vi "Update Clock Map.vi"(6 "Name":string, 7 "Reset":bool, 8 "error in (no error)":errorcluster, 9 "ClockID":u8, 10 "Timestamp Pair":T1, 11 "Clock History Map in":T3) -> (0 "error out":errorcluster, 3 "Clock History Map out":map{u8, T2}(c390))   [LabVIEW 2021, in "Time_CIF_U.lvlib"]
uses:
  Time_CIF_U.lvlib
  Typedef/Clock History Map.ctl
  Typedef/Clock History.ctl
  Typedef/Timestamp Pair.ctl
  Typedef/Errors.ctl
  <vilib>/Utility/miscctls.llb/LVMapReplaceAction.ctl
  <vilib>/Analysis/6fits.llb/Curve Fitting Criteria.ctl
  Errors/Append Error Location.vi
  <vilib>/Analysis/3filter.llb/Savitzky-Golay Filter.vi
  <vilib>/Analysis/3filter.llb/Savitzky-Golay Filter (DBL).vi
  <vilib>/Analysis/baseanly.llb/Std Deviation and Variance.vi
  <vilib>/Analysis/NI_AALPro.lvlib
  DataTypes/DataTypes_CIF_U.lvlib
panel:
  out "Slope":dbl
  out "XY Graph":cluster{i64[], i64[]}[](graph)
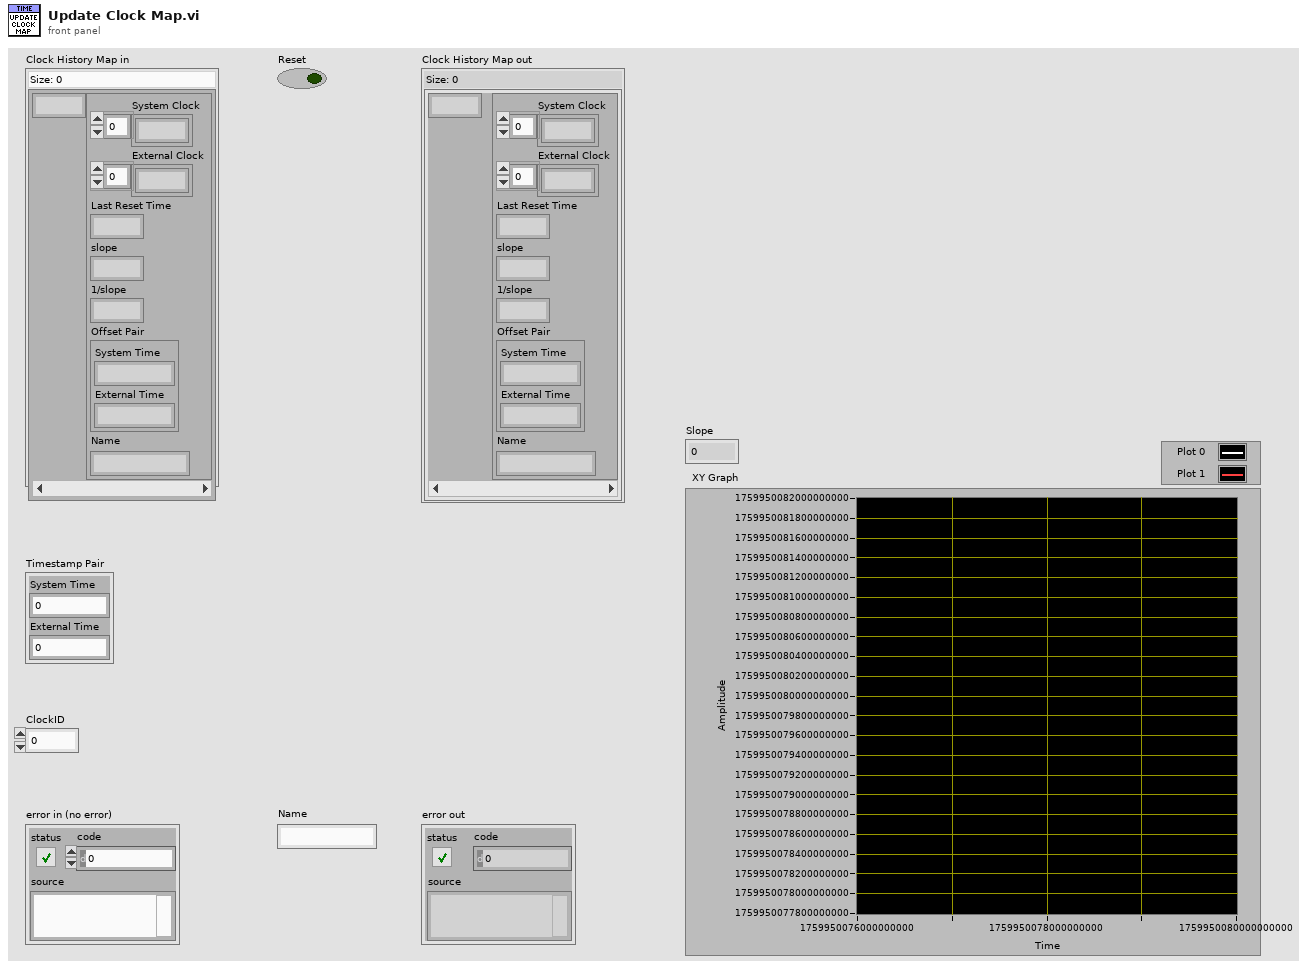
[diagram p1: front panel]
types:
  T1 = typedef "Time_CIF_U.lvlib/Timestamp Pair.ctl" = cluster{"System Time":i64, "External Time":i64}
  T2 = typedef "Time_CIF_U.lvlib/Clock History.ctl" = cluster{"System Clock":i64[], "External Clock":i64[], "Last Reset Time":i64, "slope":dbl, "1/slope":dbl, "Offset Pair":T1, "Name":string}
  T3 = typedef "Time_CIF_U.lvlib/Clock History Map.ctl" = map{u8, T2}
  T4 = typedef "Time_CIF_U.lvlib/Errors.ctl" = enum16{"Clock ID Match", "Invalid Clock ID", "Long Sleep"}
  T5 = typedef "LVMapReplaceAction.ctl" = enum32{"Modify Entry only if found", "Add or Modify Entry", "Delete Entry"}
  T6 = typedef "NI_AALPro.lvlib/Curve Fitting Criteria.ctl" = u16
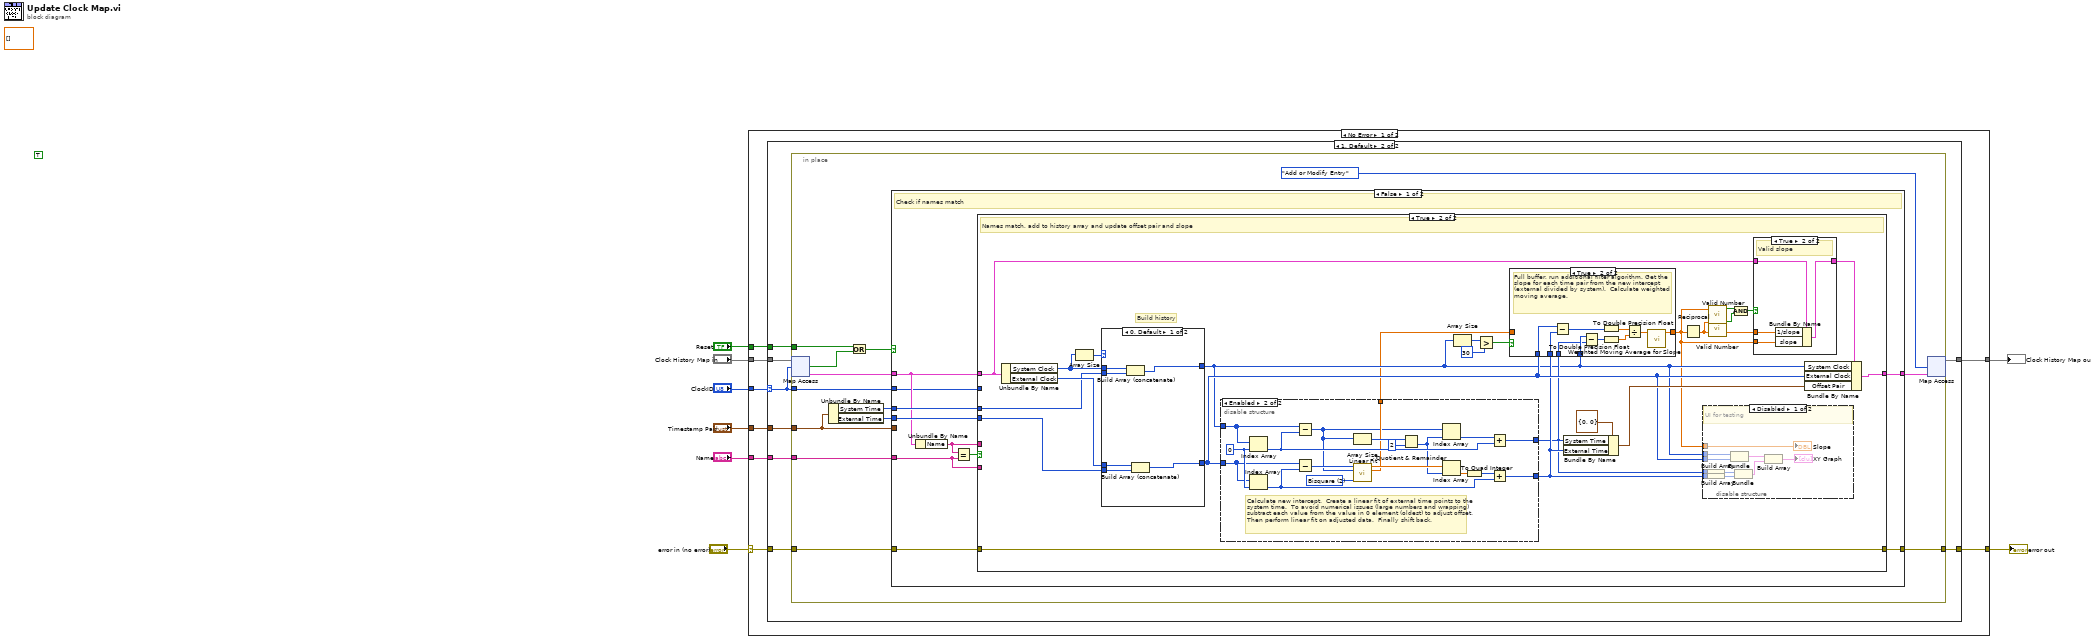
[diagram p0: block diagram]
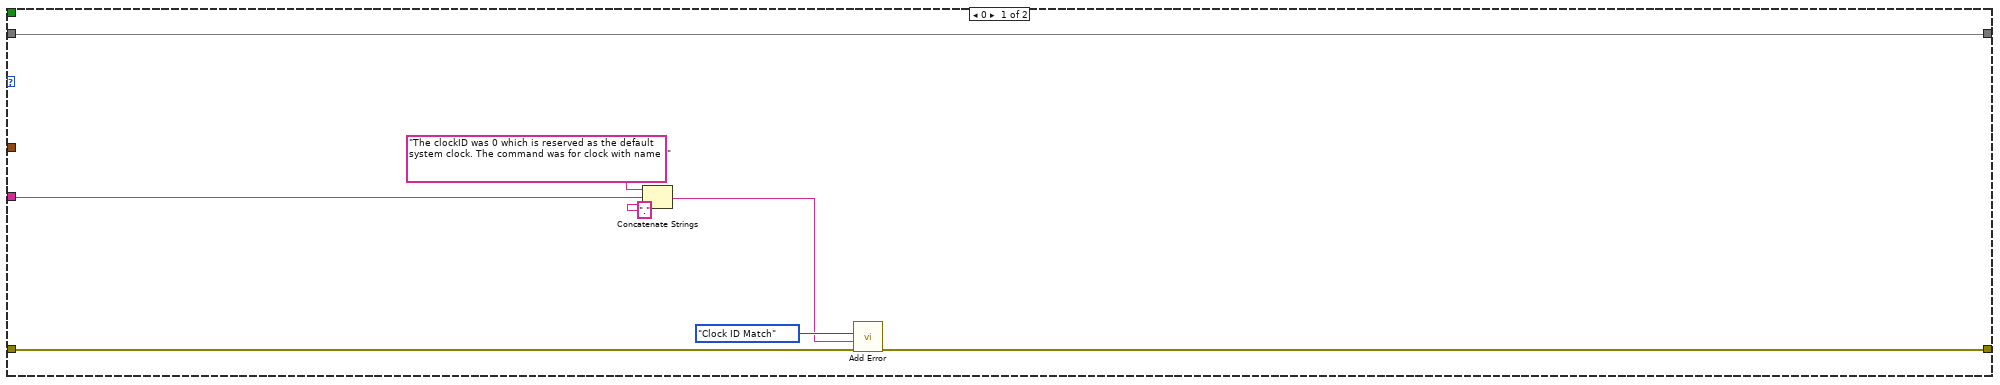
[diagram p2: hidden frame]
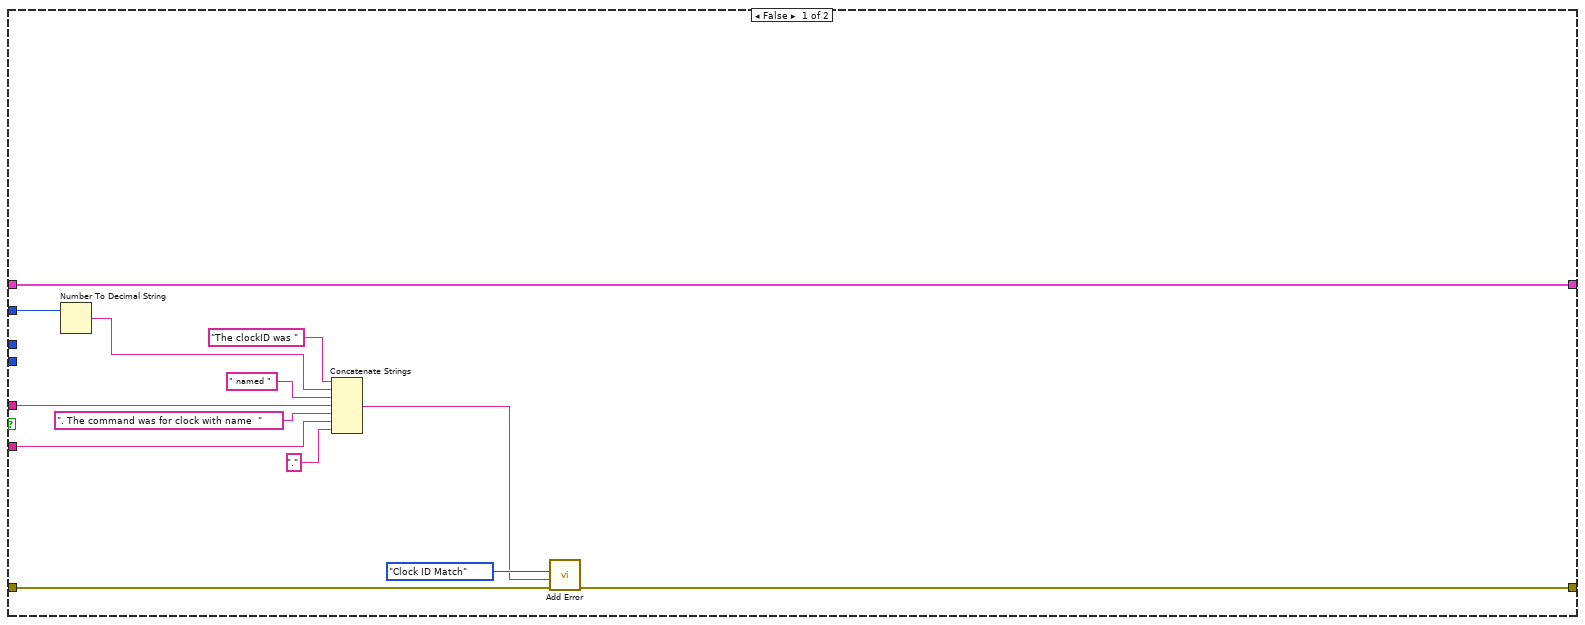
[diagram p3: hidden frame]
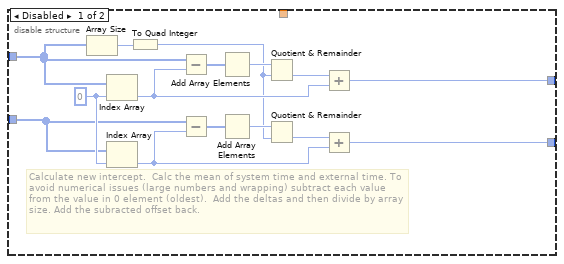
[diagram p6: hidden frame]
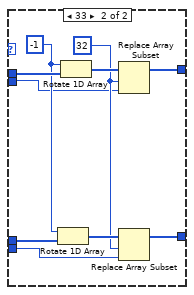
[diagram p8: hidden frame]
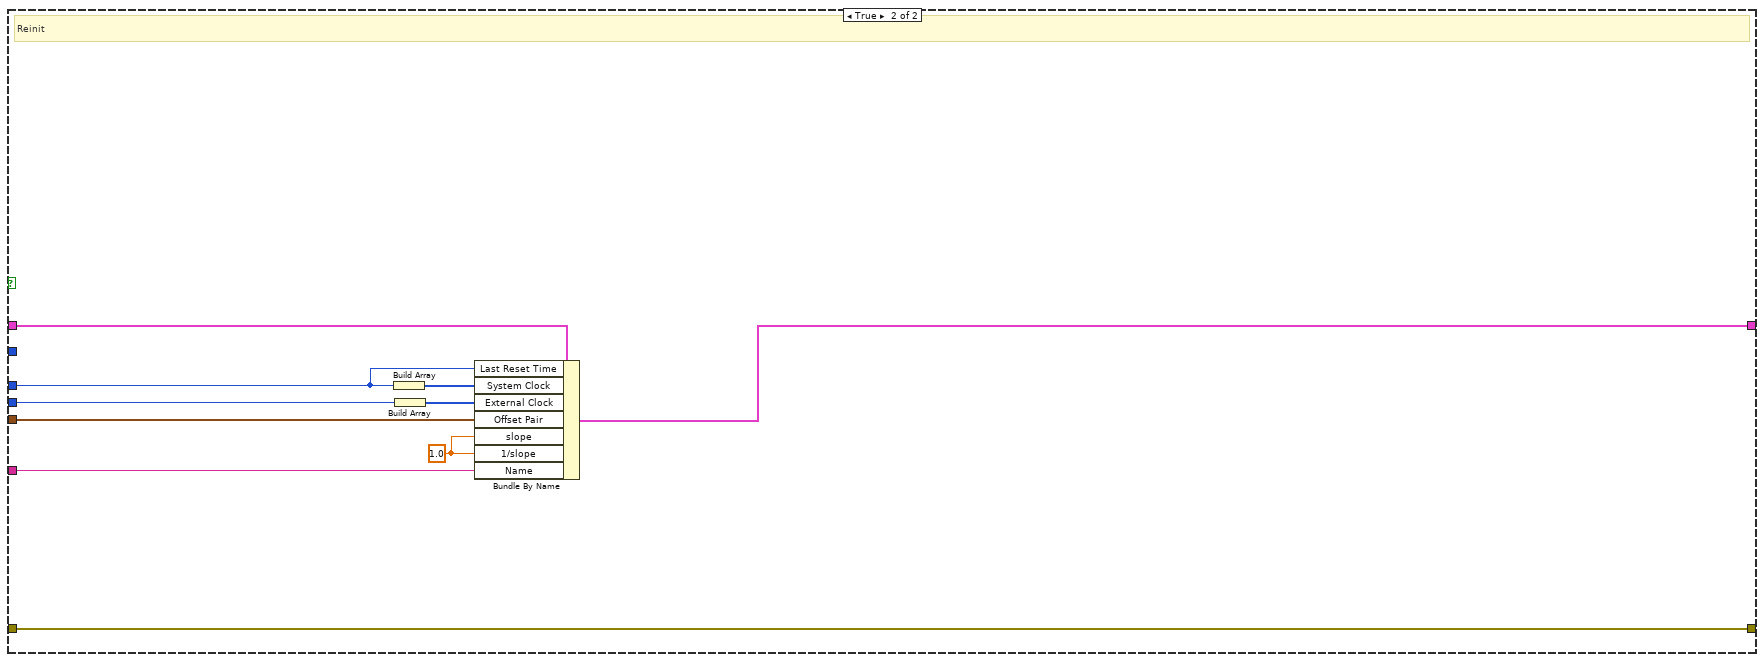
[diagram p9: hidden frame]
diagram:
  (unwired) TRUE
  (unwired) dbl[][] []
  n1 = case shown="No Error" "error in (no error)" {
    selector: "error in (no error)" -> [w10 w178]
    tunnel: "Clock History Map in" -> [w16 w179]
    tunnel: "Timestamp Pair" -> [w15 _]
    tunnel: "Reset" -> [w14 _]
    tunnel: [w13 w179] -> w5
    tunnel: "Name" -> [w12 _]
    tunnel: [w11 w178] -> w3
    tunnel: "ClockID" -> [w9 _]
    frame No Error {
      n2 = case shown="1, Default" w9 {
        selector: w9 -> [_ w25]
        tunnel: w16 -> [w19 w32]
        tunnel: w15 -> [_ w31]
        tunnel: w14 -> [_ w30]
        tunnel: [w19 w29] -> w13
        tunnel: w12 -> [w17 w28]
        tunnel: [w20 w27] -> w11
        tunnel: w10 -> [w21 w26]
        frame 0 {
          n3 = Concatenate Strings("The clockID was 0 which is reserved as the default system clock. The command was for clock with name  " ("string"), w17, "." ("string")) -> (w22:string)
          n4 = call "Add Error.vi"("error in (no error)"=w21, "String to Append"=w22, "Error"=Errors."Clock ID Match") -> ("error out"=w20:errorcluster)  [unwired: 8 in]
        }
        frame 1, Default {
          n5 = in-place {
            in-place-border: w31 -> [w38]
            in-place-border: w30 -> [w44]
            in-place-border: w28 -> [w36]
            in-place-border: w26 -> [w35]
            in-place-border: [w34] -> w27
            in-place-border: w25 -> [w33]
            n6 = in-place-map #1(w32, w25) -> (w37:T2, w45:bool)  [unwired: 1 in]
            n7 = Unbundle By Name(w38) -> ("System Time"=w40:i64, "External Time"=w39:i64)
            n8 = Or(x=w44, y=w45) -> (x .or. y?=w43:bool)
            n9 = case shown="False" w43 {
              tunnel: w37 -> [w52 w177]
              tunnel: [w53 w174] -> w42
              tunnel: w40 -> [w55 w168]
              tunnel: w39 -> [w54 w173]
              tunnel: w38 -> [_ w172]
              tunnel: w36 -> [w48 w171]
              tunnel: w35 -> [w50 w170]
              tunnel: [w49 w170] -> w34
              tunnel: w33 -> [w47 _]
              frame False {
                # "Check if names match"
                n10 = Unbundle By Name(w52) -> ("Name"=w46:string)
                n11 = Equal?(x=w46, y=w48) -> (x = y?=w51:bool)
                n12 = case shown="True" w51 {
                  tunnel: w55 -> [_ w89]
                  tunnel: w54 -> [_ w88]
                  tunnel: [w68 w84] -> w53
                  tunnel: w52 -> [w68 w83]
                  tunnel: w50 -> [w59 w82]
                  tunnel: [w58 w82] -> w49
                  tunnel: w48 -> [w60 _]
                  tunnel: w47 -> [w67 _]
                  tunnel: w46 -> [w61 _]
                  frame False {
                    n13 = Number To Decimal String(number=w67) -> (decimal integer string=w62:string)  [unwired: 1 in]
                    n14 = Concatenate Strings("The clockID was " ("string"), w62, " named " ("string"), w61, ". The command was for clock with name  " ("string"), w60, "." ("string")) -> (w56:string)
                    n15 = call "Add Error.vi"("error in (no error)"=w59, "String to Append"=w56, "Error"=Errors."Clock ID Match") -> ("error out"=w58:errorcluster)  [unwired: 8 in]
                  }
                  frame True {
                    # "Build history"
                    # "Names match, add to history array and update offset pair and slope"
                    n16 = Unbundle By Name(w83) -> ("System Clock"=w90:i64[], "External Clock"=w91:i64[])
                    n17 = Array Size(array=w90) -> (size(s)=w92:i32)
                    n18 = case shown="0, Default" w92 {
                      tunnel: w91 -> [w155 w167]
                      tunnel: w90 -> [w157 w166]
                      tunnel: [w156 w161] -> w77
                      tunnel: [w154 w160] -> w80
                      tunnel: w89 -> [w153 w158]
                      tunnel: w88 -> [w152 w159]
                      frame 0, Default {
                        n19 = Build Array (concatenate)(w157, w153) -> (w156:i64[])
                        n20 = Build Array (concatenate)(w155, w152) -> (w154:i64[])
                      }
                      frame 33 {
                        w162 = 32 ("index")
                        w165 = -1 ("n")
                        n21 = Rotate 1D Array(1:w167, 2:w165) -> (0:w164:i64[])
                        n22 = Rotate 1D Array(1:w166, 2:w165) -> (0:w163:i64[])
                        n23 = Replace Array Subset(array=w163, new element=w158, index=w162) -> (w161:i64[])
                        n24 = Replace Array Subset(array=w164, new element=w159, index=w162) -> (w160:i64[])
                      }
                    }
                    n25 = disable-structure shown="Enabled" {
                      disable-tunnel: [w118 w144] -> w78
                      disable-tunnel: [w117 w143] -> w79
                      disable-tunnel: w77 -> [w116 w142]
                      disable-tunnel: w80 -> [w115 w141]
                      disable-tunnel: [_ w134] -> w73
                      frame Disabled {
                        w122 = 0 ("index")
                        # "Calculate new intercept.  Calc the mean of system time and external time. To avoid numerical issues (large numbers and wrapping) subtract each value from the value in 0 element (oldest).  Add the deltas and then divide by array size. Add the subracted offset back."
                        n26 = Array Size(array=w116) -> (size(s)=w121:i32)
                        n27 = Index Array(array=w116, index=w122) -> (element=w120:i64)
                        n28 = Index Array(array=w115, index=w122) -> (element=w114:i64)
                        n29 = To Quad Integer(1:w121) -> (0:w119:i64)
                        n30 = Subtract(x=w116, y=w120) -> (x-y=w128:i64[])
                        n31 = Subtract(x=w115, y=w114) -> (x-y=w123:i64[])
                        n32 = Add Array Elements(numeric array=w128) -> (sum=w127:i64)
                        n33 = Add Array Elements(numeric array=w123) -> (sum=w124:i64)
                        n34 = Quotient & Remainder(x=w127, y=w119) -> (floor(x/y)=w126:i64)  [unwired: 1 out]
                        n35 = Quotient & Remainder(x=w124, y=w119) -> (floor(x/y)=w125:i64)  [unwired: 1 out]
                        n36 = Add(x=w126, y=w120) -> (x+y=w118:i64)
                        n37 = Add(x=w125, y=w114) -> (x+y=w117:i64)
                      }
                      frame Enabled {
                        w135 = T6 2 items=["Least Square", "Least Absolute Residual", "Bisquare"] ("method")
                        w146 = 0 ("index")
                        # "Calculate new intercept.  Create a linear fit of external time points to the system time.  To avoid numerical issues (large numbers and wrapping) subtract each value from the value in 0 element (oldest) to adjust offset.  Then perform linear fit on adjusted data.  Finally shift back."
                        n38 = Index Array(array=w142, index=w146) -> (element=w145:i64)
                        n39 = Index Array(array=w141, index=w146) -> (element=w129:i64)
                        n40 = Subtract(x=w142, y=w145) -> (x-y=w132:i64[])
                        n41 = Subtract(x=w141, y=w129) -> (x-y=w133:i64[])
                        n42 = call <vilib>:"Linear Fit.vi"("Y"=w133, "X"=w132, "method"=w135) -> ("Best Linear Fit"=w139:dbl[], "slope"=w134:dbl)  [unwired: 8 in, 3 out]
                        n43 = Array Size(array=w132) -> (size(s)=w140:i32)
                        n44 = Quotient & Remainder(x=w140, y=2) -> (floor(x/y)=w138:i32)  [unwired: 1 out]
                        n45 = Index Array(array=w132, index=w138) -> (element=w130:i64)
                        n46 = Index Array(array=w139, index=w138) -> (element=w137:dbl)
                        n47 = To Quad Integer(1:w137) -> (0:w131:i64)
                        n48 = Add(x=w130, y=w145) -> (x+y=w144:i64)
                        n49 = Add(x=w131, y=w129) -> (x+y=w143:i64)
                      }
                    }
                    n50 = Array Size(array=w77) -> (size(s)=w76:i32)
                    n51 = Greater?(x=w76, y=30) -> (0:w74:bool)
                    n52 = case shown="True" w74 {
                      tunnel: [w103 w108] -> w72
                      tunnel: w77 -> [_ w107]
                      tunnel: w80 -> [_ w106]
                      tunnel: w79 -> [_ w105]
                      tunnel: w78 -> [_ w104]
                      tunnel: w73 -> [w103 _]
                      frame False {
                        # "Buffer not full don't apply additional slope filter"
                      }
                      frame True {
                        # "Full buffer, run additional filter algorithm. Get the slope for each time pair from the new intercept (external divided by system).  Calculate weighted moving average."
                        n53 = Subtract(x=w106, y=w105) -> (x-y=w109:i64[])
                        n54 = Subtract(x=w107, y=w104) -> (x-y=w110:i64[])
                        n55 = To Double Precision Float(number=w109) -> (double precision float=w111:dbl[])
                        n56 = To Double Precision Float(number=w110) -> (double precision float=w112:dbl[])
                        n57 = Divide(x=w111, y=w112) -> (x/y=w113:dbl[])
                        n58 = call "Weighted Moving Average for Slope.vi"("Slopes"=w113) -> ("Slope"=w108:dbl)  [unwired: 10 in]
                      }
                    }
                    n59 = Bundle By Name(cluster=T1 {"System Time"=0, "External Time"=0} ("Offset Pair"), "System Time"=w78, "External Time"=w79) -> (w86:T1)
                    n60 = Reciprocal(x=w72) -> (1/x=w69:dbl)
                    n61 = disable-structure shown="Disabled" {
                      disable-tunnel: w80 -> [w102 _]
                      disable-tunnel: w79 -> [w96 _]
                      disable-tunnel: w78 -> [w95 _]
                      disable-tunnel: w77 -> [w94 _]
                      disable-tunnel: w72 -> [w93 _]
                      frame Disabled {
                        # "UI for testing"
                        n62 = Build Array(w95) -> (w98:i64[])
                        n63 = Build Array(w96) -> (w97:i64[])
                        n64 = Bundle(w94, w102) -> (w101:cluster{i64[], i64[]})  [unwired: 1 in]
                        n65 = Bundle(w98, w97) -> (w100:cluster{i64[], i64[]})  [unwired: 1 in]
                        n66 = Build Array(w101, w100) -> (→"XY Graph":cluster{i64[], i64[]}[])
                        "Slope" <- w93
                      }
                      frame Enabled {
                      }
                    }
                    n67 = call "Valid Number.vi"("Number"=w72) -> ("Valid"=w71:bool)  [unwired: 4 in]
                    n68 = call "Valid Number.vi"("Number"=w69) -> ("Valid"=w70:bool)  [unwired: 4 in]
                    n69 = Compound Arithmetic op=AND(w71, w70) -> (w81:bool)
                    n70 = case shown="True" w81 {
                      tunnel: w72 -> [_ w149]
                      tunnel: w83 -> [w147 w151]
                      tunnel: [w147 w150] -> w85
                      tunnel: w69 -> [_ w148]
                      frame False {
                        # "NaN, don't update slope"
                      }
                      frame True {
                        # "Valid slope"
                        n71 = Bundle By Name(cluster=w151, "1/slope"=w148, "slope"=w149) -> (w150:T2)
                      }
                    }
                    n72 = Bundle By Name(cluster=w85, "System Clock"=w77, "External Clock"=w80, "Offset Pair"=w86) -> (w84:T2)
                  }
                }
              }
              frame True {
                w169 = 1.0 ("slope")
                # "Reinit"
                n73 = Build Array(w168) -> (w176:i64[])
                n74 = Build Array(w173) -> (w175:i64[])
                n75 = Bundle By Name(cluster=w177, "Last Reset Time"=w168, "System Clock"=w176, "External Clock"=w175, "Offset Pair"=w172, "slope"=w169, "1/slope"=w169, "Name"=w171) -> (w174:T2)
              }
            }
            n76 = in-place-map #1(w42, LVMapReplaceAction."Add or Modify Entry" ("action")) -> (w29:T3)  [unwired: 2 out]
          }
        }
      }
    }
    frame Error {
    }
  }
  "Clock History Map out" <- w5
  "error out" <- w3
